vi "Measure.vi"(8 "error in":errorcluster, 9 "gRPCid in":T1, 10 "pin map id":string, 11 "measurement configuration":T3) -> (0 "error out":errorcluster, 2 "gRPCid out":u64, 3 "measurement results":T2)   [LabVIEW 2021, in "Measurement Client Template.lvlib"]
doc: "Invoke the Measurement Logic and get the results"
uses:
  Measurement Client Template.lvlib
  controls/Measurement Configuration.ctl
  controls/Measurement Results.ctl
  <vilib>/gRPC/LabVIEW gRPC Library/Shared/grpcId.ctl
  <vilib>/gRPC/Generated APIs/ni/measurementlink/measurement/v2/Measurement Service Client/RPC Messages/ni_measurementlink_measurement_v2_MeasureRequest.ctl
  <vilib>/gRPC/Generated APIs/ni/measurementlink/measurement/v2/Measurement Service Client/RPC Messages/google_protobuf_Any.ctl
  <vilib>/gRPC/Generated APIs/ni/measurementlink/measurement/v2/Measurement Service Client/RPC Messages/ni_measurementlink_PinMapContext.ctl
  c8e7d04f-3e50-4eba-9c41-e335012f285e.vi
  233c5f21-7ff6-44c7-820f-94d9e0a33a0d.vi
  <vilib>/gRPC/LabVIEW gRPC Library/Server API/Translate Protobuf Error.vi
  <vilib>/AdvancedString/1D String Array to Delimited String.vi
  <vilib>/gRPC/LabVIEW gRPC Library/Server API/Server/Get Server DLL Path.vi
  <vilib>/gRPC/Generated APIs/ni/measurementlink/measurement/v2/Measurement Service Client/Measurement Service Client.lvlib
  <vilib>/gRPC/LabVIEW gRPC Library/grpc-lvsupport-release.lvlib
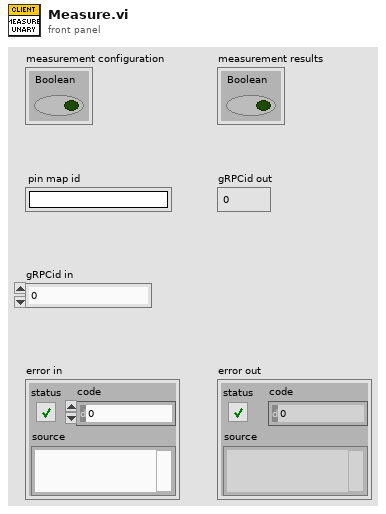
[diagram p1: front panel]
types:
  T1 = typedef "grpc-lvsupport-release.lvlib/grpcId.ctl" = u64
  T2 = typedef "Measurement Client Template.lvlib/Measurement Results.ctl" = cluster{"Boolean":bool}
  T3 = typedef "Measurement Client Template.lvlib/Measurement Configuration.ctl" = cluster{"Boolean":bool}
  T4 = typedef "ni.measurementlink.measurement.v2.api.lvlib/Measurement Service Client.lvlib/ni_measurementlink_measurement_v2_MeasureRequest.ctl" = cluster{"configuration_parameters":T5, "pin_map_context":T6}
  T5 = typedef "ni.measurementlink.measurement.v2.api.lvlib/Measurement Service Client.lvlib/google_protobuf_Any.ctl" = cluster{"type_url":string, "value":u8[]}
  T6 = typedef "ni.measurementlink.measurement.v2.api.lvlib/Measurement Service Client.lvlib/ni_measurementlink_PinMapContext.ctl" = cluster{"pin_map_id":string, "sites":i32[]}
  T7 = typedef "grpc-lvsupport-release.lvlib/Any.ctl" = cluster{"Type Url":string, "Bytes":u8[]}
  T8 = typedef "ni.measurementlink.measurement.v2.api.lvlib/Measurement Service Client.lvlib/ni_measurementlink_measurement_v2_MeasureResponse.ctl" = cluster{"outputs":T5}
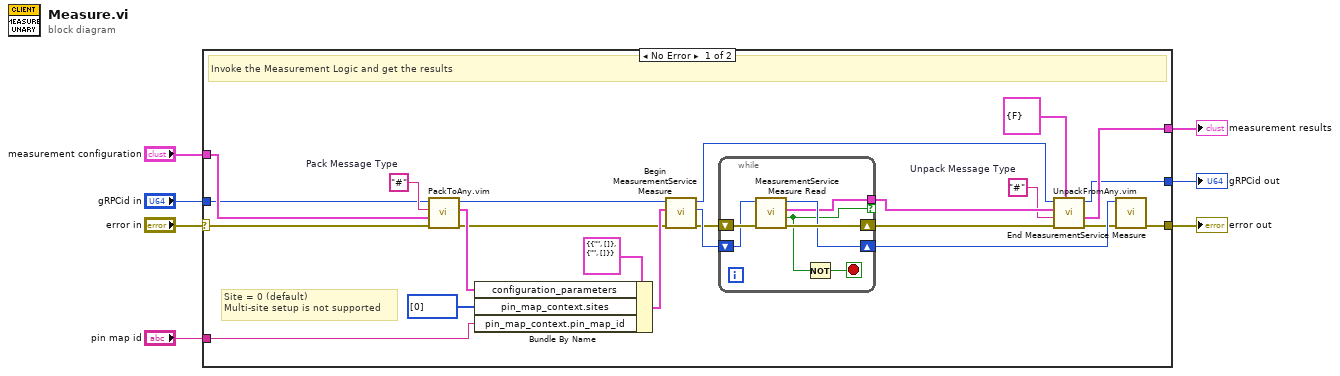
[diagram p0: block diagram]
diagram:
  n1 = case shown="No Error" "error in" {
    selector: "error in" -> [w12 w39]
    tunnel: "measurement configuration" -> [w29 _]
    tunnel: "pin map id" -> [w26 _]
    tunnel: [w24 _] -> w5
    tunnel: [w20 w39] -> w4
    tunnel: "gRPCid in" -> [w11 w38]
    tunnel: [w10 w38] -> w1
    frame No Error {
      w9 = "#"  # Unpack Message Type
      w30 = "#"  # Pack Message Type
      # "Site = 0 (default)\nMulti-site setup is not supported"
      # "Invoke the Measurement Logic and get the results"
      n2 = call "PackToAny.vim"("error in"=w12, "Data To Pack"=w29, "Message Type"=w30, "gRPCid in"=w11) -> ("error out"=w14:errorcluster, "Any"=w15:T7, "gRPCid out"=w25:u64)  [unwired: 5 in]
      n3 = Bundle By Name(cluster=T4 {"configuration_parameters"={"type_url"="", "value"=[]}, "pin_map_context"={"pin_map_id"="", "sites"=[]}} ("Request Data"), "configuration_parameters"=w15, "pin_map_context.sites"=i32[] [0], "pin_map_context.pin_map_id"=w26) -> (w16:T4)
      n4 = call <vilib>:"Begin MeasurementService Measure.vi"("error in"=w14, "Request Data"=w16, "gRPC ID"=w25) -> ("error out"=w17:errorcluster, "Call Id Out"=w21:T1, "gRPC ID out"=w23:T1)  [unwired: 6 in]
      n5 = while {
        shift-right: [w36] -> w18
        shift-left: w17 -> [w37]
        shift-right: [w34] -> w22
        shift-left: w21 -> [w35]
        tunnel: [w32] -> w28 if=w31
        stop <- w33 stop-if-true
        n6 = call <vilib>:"MeasurementService Measure Read.vi"("error in"=w37, "Call ID in"=w35) -> ("error out"=w36:errorcluster, "Success"=w31:bool, "Response Data"=w32:T8, "Call ID"=w34:T1)  [unwired: 6 in]
        n7 = Not(x=w31) -> (.not. x?=w33:bool)
      }
      n8 = call "UnpackFromAny.vim"("Data Type"=T2 {"Boolean"=FALSE} ("measurement results"), "error in"=w18, "Message Type"=w9, "Any"=w28, "gRPCid in"=w23) -> ("error out"=w19:errorcluster, "Unpacked Value"=w24:T2, "gRPCid out"=w10:u64)  [unwired: 4 in]
      n9 = call <vilib>:"End MeasurementService Measure.vi"("error in"=w19, "Call ID in"=w22) -> ("error out"=w20:errorcluster)  [unwired: 8 in, 1 out]
    }
    frame Error {
      # "Pass"
    }
  }
  "measurement results" <- w5
  "gRPCid out" <- w1
  "error out" <- w4
